vi "Find Friends.vi"(11 "Square in":refnum<class "Square.lvclass">) -> (2 "Friend Directions":T1[](array[typedef]))   [LabVIEW 2020, in "SquareBattle.lvlib" / "Square.lvclass"]
uses:
  Square.lvclass
  Direction.ctl
  Square.lvclass/Square.ctl
  SquareBattle.lvlib
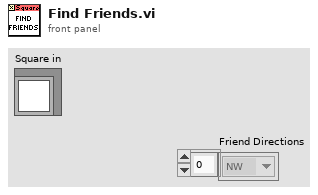
[diagram p1: front panel]
types:
  T1 = typedef "SquareBattle.lvlib/Direction.ctl" = enum16{"NW", "N", "NE", "E", "SE", "S", "SW", "W"}
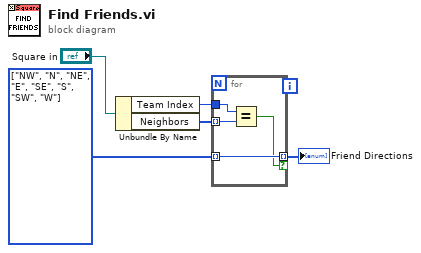
[diagram p0: block diagram]
diagram:
  w2 = T1[] [enum."NW", enum."N", enum."NE", enum."E", enum."SE", enum."S", enum."SW", enum."W"] items=["NW", "N", "NE", "E", "SE", "S", "SW", "W"] ("Enemy Directions")
  n1 = Unbundle By Name("Square in") -> ("Team Index"=w4:i32, "Neighbors"=w3:i32[])
  n2 = for {
    tunnel: w4 -> [w8]
    tunnel: w3 -> [w7] mode=indexing
    tunnel: w2 -> [w9] mode=indexing
    tunnel: [w9] -> w1 mode=indexing if=w6
    n3 = Equal?(x=w8, y=w7) -> (x = y?=w6:bool)
  }
  "Friend Directions" <- w1
